vi "FTW-Endpoint-Multipart-Receive.vi"(0 "FTW Endpoint":refnum<class "FTW-Endpoint-TCP.lvclass">, 5 "Timeout":i32 format="%dmsec", 11 "error in":errorcluster) -> (4 "FTW Endpoint out":refnum<class "FTW-Endpoint-TCP.lvclass">, 6 "Message Received":T1, 8 "Timed out?":bool, 15 "error out":errorcluster)   [LabVIEW 2013, in "FTW-Endpoint-TCP.lvclass"]
uses:
  FTW-Endpoint-TCP.lvclass
  Payload/FTW-MessagePayload.ctl
  FTW-Endpoint-TCP.lvclass/FTW-Endpoint-TCP.ctl
  Error/FTW-ERR-Clear.vi
panel:
  # "Inputs"
  # "Outputs"
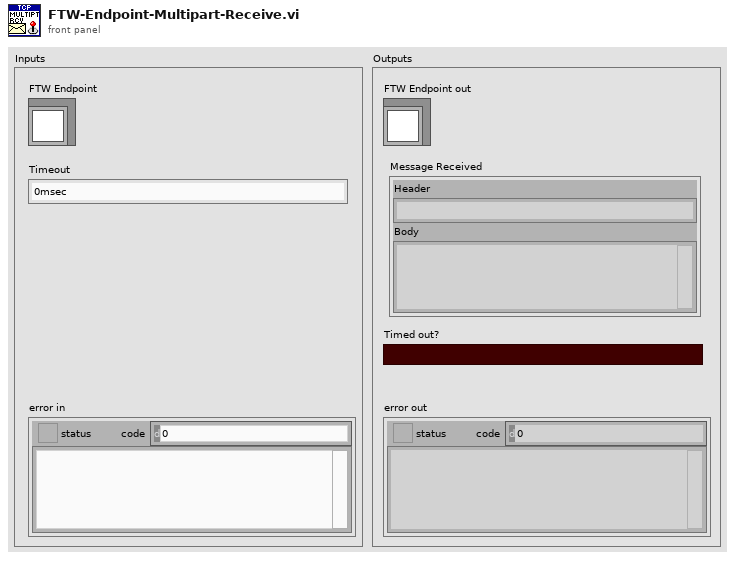
[diagram p1: front panel]
types:
  T1 = typedef "FTW-MessagePayload.ctl" = cluster{"Header":string, "Body":string, "FTW: Sender Identity":string, "FTW: Reply Address":string, "FTW: Reply Error":errorcluster}
  T2 = enum16{"Standard", "Buffered", "CRLF", "Immediate"}
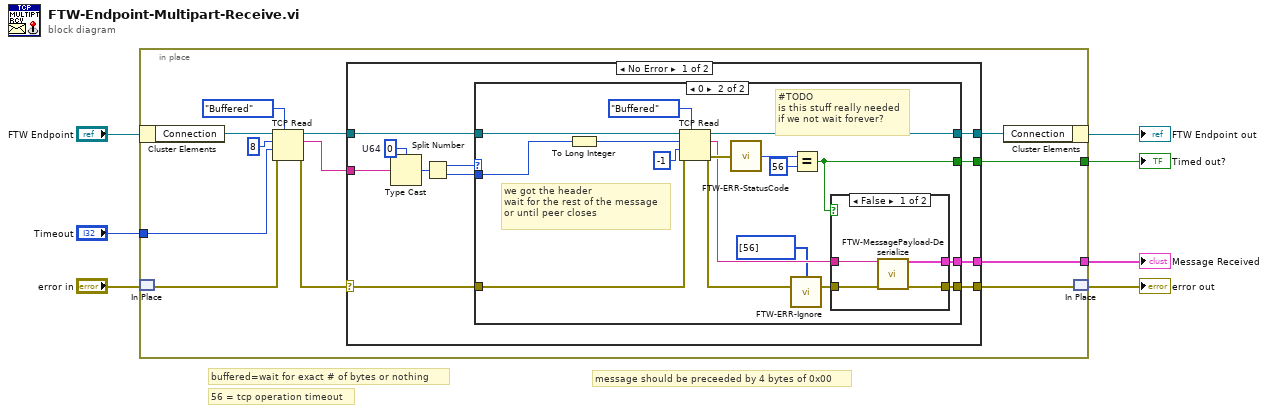
[diagram p0: block diagram]
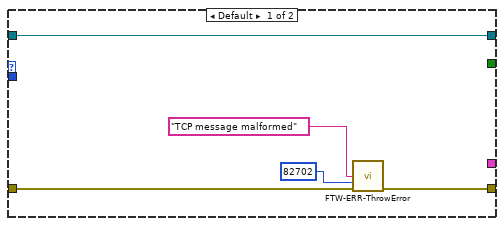
[diagram p2: hidden frame]
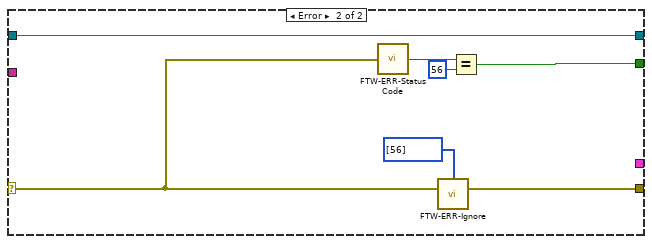
[diagram p4: hidden frame]
diagram:
  # "message should be preceeded by 4 bytes of 0x00"
  # "56 = tcp operation timeout"
  # "buffered=wait for exact # of bytes or nothing"
  n1 = in-place {
    in-place-border: "Timeout" -> [w10]
    in-place-border: [w13] -> w4
    in-place-border: [w12] -> w3
    n2 = in-place-cluster #1("FTW Endpoint") -> ("Connection"=w15:refnum<k5>)
    n3 = in-place-match #2("error in") -> (w9:errorcluster)
    n4 = TCP Read(connection ID=w15, bytes to read=8, error in (no error)=w9, 7:T2."Buffered" ("mode (standard)"), 9:w10) -> (connection ID out=w17:refnum<k5>, data out=w11:string, error out=w18:errorcluster)
    n5 = case shown="No Error" w18 {
      selector: w18 -> [w22 w59]
      tunnel: w17 -> [w30 w57]
      tunnel: [w29 w57] -> w14
      tunnel: [w28 w58] -> w8
      tunnel: [w27 _] -> w13
      tunnel: [w26 w60] -> w12
      tunnel: w11 -> [w23 _]
      frame No Error {
        w25 = u64 0  # U64
        n6 = Type Cast(type=w25, x=w23) -> (*(type *) &x=w24:u64)
        n7 = Split Number(x=w24) -> (hi(x)=w20:u32, lo(x)=w21:u32)
        n8 = case shown="0" w20 {
          tunnel: w30 -> [w35 w51]
          tunnel: [w35 w50] -> w29
          tunnel: [w33 w49] -> w28
          tunnel: [_ w46] -> w27
          tunnel: [_ w43] -> w26
          tunnel: w22 -> [w34 w39]
          tunnel: w21 -> [_ w37]
          frame Default {
            n9 = call "FTW-ERR-ThrowError.vi"("Error Message"="TCP message malformed", "Error Code"=82702, "error in"=w34) -> ("error out"=w33:errorcluster)  [unwired: 12 in]
          }
          frame 0 {
            # "#TODO\nis this stuff really needed\nif we not wait forever?"
            # "we got the header\nwait for the rest of the message\nor until peer closes"
            n10 = To Long Integer(number=w37) -> (32bit integer=w36:i32)
            n11 = TCP Read(connection ID=w51, bytes to read=w36, error in (no error)=w39, 7:T2."Buffered" ("mode (standard)"), 9:-1) -> (connection ID out=w50:refnum<k5>, data out=w45:string, error out=w48:errorcluster)
            n12 = call "FTW-ERR-StatusCode.vi"("error to check"=w48) -> ("Code"=w47:i32)
            n13 = call "FTW-ERR-Ignore.vi"("Codes to filter"=i32[] [56], "error to filter"=w48) -> ("filtered error"=w42:errorcluster)  [unwired: 13 in]
            n14 = Equal?(x=w47, y=56 ("x")) -> (x = y?=w43:bool)
            n15 = case shown="False" w43 {
              tunnel: [w55 w56] -> w49
              tunnel: w42 -> [w54 w56]
              tunnel: [w53 _] -> w46
              tunnel: w45 -> [w52 _]
              frame False {
                n16 = call "FTW-MessagePayload-Deserialize.vi"("Serialized Message String"=w52, "error in"=w54) -> ("Message"=w53:T1, "error out"=w55:errorcluster)  [unwired: 12 in]
              }
              frame True {
              }
            }
          }
        }
      }
      frame Error {
        n17 = call "FTW-ERR-StatusCode.vi"("error to check"=w59) -> ("Code"=w63:i32)
        n18 = call "FTW-ERR-Ignore.vi"("Codes to filter"=i32[] [56], "error to filter"=w59) -> ("filtered error"=w58:errorcluster)  [unwired: 13 in]
        n19 = Equal?(x=w63, y=56 ("x")) -> (x = y?=w60:bool)
      }
    }
    n20 = in-place-cluster #1("Connection"=w14) -> (→"FTW Endpoint out":refnum<class "FTW-Endpoint-TCP.lvclass">)
    n21 = in-place-match #2(w8) -> (→"error out":errorcluster)
  }
  "Message Received" <- w4
  "Timed out?" <- w3
